vi "BC Verify Message Command.vi"(5 "Instruction ID":i32, 6 "Cmd Address":u16 format="%04x", 7 "Target IC (1-8)":u8, 8 "error in (no error)":errorcluster, 9 "Transmit?":bool, 10 "RT-RT?":bool, 11 "Bus Controller in":refnum<class "Bus Controller.lvclass">) -> (0 "error out":errorcluster, 3 "Bus Controller out":refnum<class "Bus Controller.lvclass">, 4 "Post-Data Address":u16 format="%04x")   [LabVIEW 2020, in "Unit Tests.lvlib" / "Bus Controller.lvclass"]
uses:
  Bus Controller.lvclass
  Bus Controller.lvclass/Bus Controller.ctl
  <vilib>/addons/_JKI Toolkits/Caraya/classes/Assert/Assert True.vi
  Dependencies/FPGA Interface/FPGA Interface.lvclass
  <vilib>/addons/_JKI Toolkits/Caraya/classes/Assert/Assert.lvclass
  <vilib>/addons/_JKI Toolkits/Caraya/classes/Test/Test.lvclass
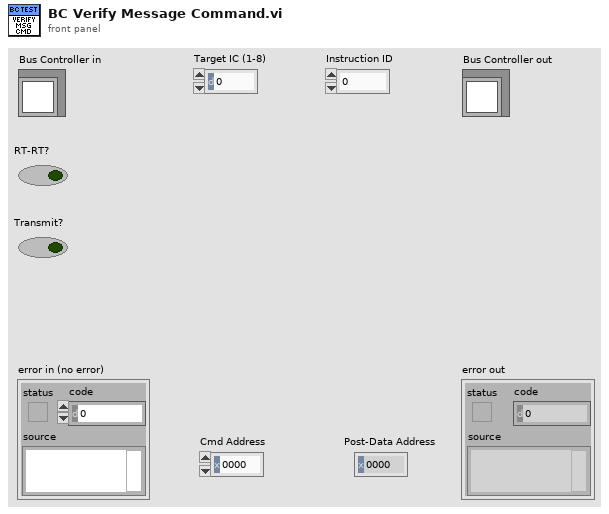
[diagram p1: front panel]
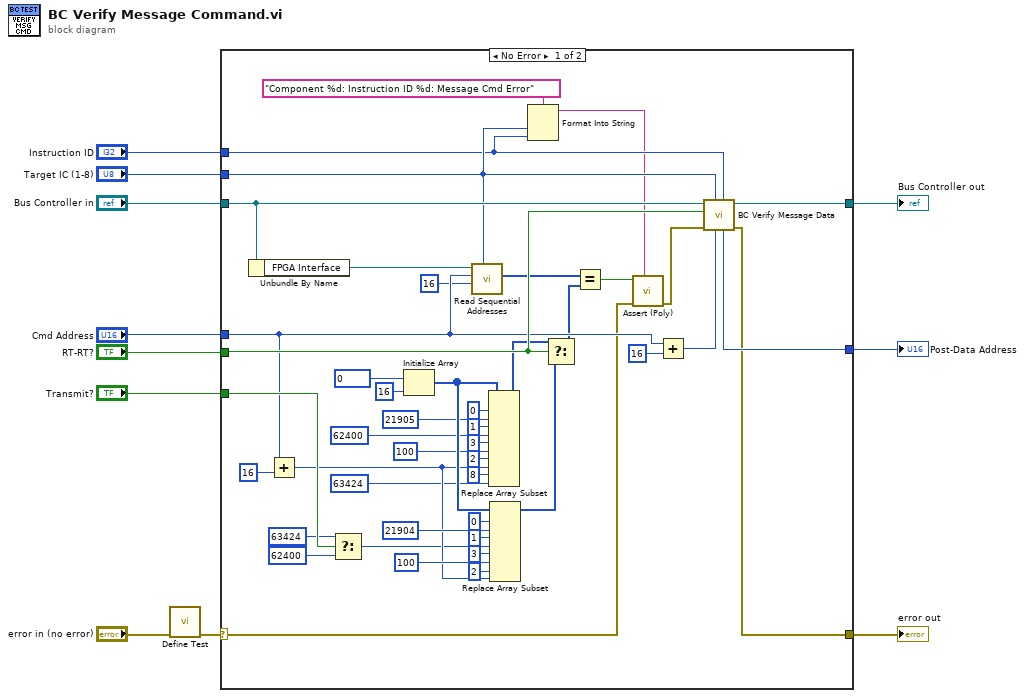
[diagram p0: block diagram]
diagram:
  n1 = call <vilib>:"Define Test.vi"("error in (no error)"="error in (no error)") -> ("error out"=w3:errorcluster)  [unwired: 9 in, 1 out]
  n2 = case shown="No Error" w3 {
    selector: w3 -> [w48 w59]
    tunnel: [w47 w59] -> w11
    tunnel: [w49 w58] -> w9
    tunnel: "Bus Controller in" -> [w55 w58]
    tunnel: "Cmd Address" -> [w51 w57]
    tunnel: "RT-RT?" -> [w54 _]
    tunnel: "Transmit?" -> [w56 _]
    tunnel: "Target IC (1-8)" -> [w53 _]
    tunnel: "Instruction ID" -> [w52 _]
    tunnel: [w50 w57] -> w1
    frame No Error {
      n3 = Unbundle By Name(w55) -> ("FPGA Interface"=w21:refnum<class "FPGA Interface.lvclass">)
      n4 = Add(x=w51, y=u16 16) -> (x+y=w26:u16)
      n5 = Select(t=u16 63424, s=w56, f=u16 62400) -> (s? t:f=w23:u16)
      n6 = Initialize Array(u16 0, 16 ("dimension size")) -> (w43:u16[])
      n7 = call-dynamic "Read Sequential Addresses.vi"("Target IC (1-8)"=w53, "Addresses to Read"=u16 16, "Starting Address"=w51, "FPGA Interface in"=w21) -> ("Data"=w19:u16[])  [unwired: 6 in, 1 out]
      n8 = Replace Array Subset(array=w43, new element #1=u16 21905, index #1=0 ("index"), new element #2=u16 62400, index #2=1 ("index"), new element #3=u16 100 ("dimension size"), index #3=3 ("index"), new element #4=w26, index #4=2 ("index"), new element #5=u16 63424, index #5=8 ("index")) -> (w44:u16[])
      n9 = Replace Array Subset(array=w43, new element #1=u16 21904, index #1=0 ("index"), new element #2=w23, index #2=1 ("index"), new element #3=u16 100 ("new element/subarray"), index #3=3 ("index"), new element #4=w26, index #4=2 ("index")) -> (w38:u16[])
      n10 = Format Into String(format string="Component %d: Instruction ID %d: Message Cmd Error" ("message (\"\")"), w53, w52) -> (resulting string=w15:string)  [unwired: 2 in, 1 out]
      n11 = Select(t=w44, s=w54, f=w38) -> (s? t:f=w18:u16[])
      n12 = Equal?(x=w19, y=w18) -> (x = y?=w17:bool)
      n13 = call-poly <vilib>:"Assert (Poly).vi"("Label"=w15, "error in (no error)"=w48, "True?"=w17) -> ("error out"=w12:errorcluster)  [unwired: 7 in, 1 out]
      n14 = Add(x=w51, y=u16 16) -> (x+y=w13:u16)
      n15 = call "BC Verify Message Data.vi"("Instruction ID"=w52, "Data Address"=w13, "Target IC (1-8)"=w53, "error in (no error)"=w12, "RT-RT?"=w54, "Bus Controller in"=w55) -> ("error out"=w47:errorcluster, "Bus Controller out"=w49:refnum<class "Bus Controller.lvclass">, "Post-Data Address"=w50:u16)  [unwired: 3 in]
    }
    frame Error {
    }
  }
  "error out" <- w11
  "Bus Controller out" <- w9
  "Post-Data Address" <- w1
